vi "TCam_Overlay.vi"(8 "error in (no error)":errorcluster, 9 "OverlayTemp?":bool, 10 "Mouse pos":cluster{"X":i32, "Y":i32}, 11 "img in":T1) -> (0 "error out":errorcluster, 3 "Image Out":T1)   [LabVIEW 2024]
uses:
  <vilib>/vision/Image Controls.llb/IMAQ Image.ctl
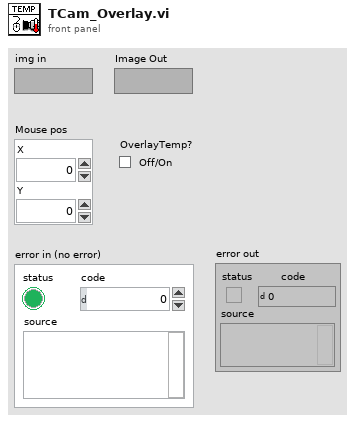
[diagram p1: front panel]
types:
  T1 = typedef "IMAQ Image.ctl" = refnum<image>
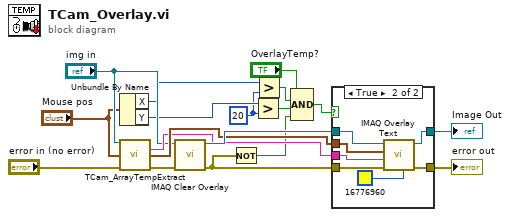
[diagram p0: block diagram]
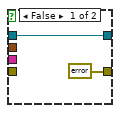
[diagram p2: hidden frame]
diagram:
  w3 = 20 ("x")
  n1 = Unbundle By Name("Mouse pos") -> ("X"=w2:i32, "Y"=w9:i32)
  n2 = call "TCam_ArrayTempExtract.vi"("img in"="img in", "Mouse pos"="Mouse pos", "error in (no error)"="error in (no error)") -> ("temp str"=w16:string, "Mouse pos dup"=w17:cluster{"X":i32, "Y":i32}, "error out"=w14:errorcluster)  [unwired: 8 in, 2 out]
  n3 = call "IMAQ Clear Overlay"("error in (no error)"=w14, "Image"="img in") -> ("error out"=w8:errorcluster, "Image Out"=w18:T1)  [unwired: 8 in]
  n4 = Not(x=w8) -> (.not. x?=w5:bool)
  n5 = Greater?(x=w9, y=w3) -> (0:w6:bool)
  n6 = Greater?(x=w2, y=w3) -> (0:w4:bool)
  n7 = Compound Arithmetic op=AND("OverlayTemp?", w4, w6, w5) -> (w7:bool)
  n8 = case shown="True" w7 {
    tunnel: w18 -> [w20 w27]
    tunnel: w8 -> [_ w26]
    tunnel: w17 -> [_ w25]
    tunnel: w16 -> [_ w24]
    tunnel: [w20 w23] -> w12
    tunnel: [errorcluster {"status"=FALSE, "code"=0, "source"=""} ("error out") w22] -> w11
    frame False {
    }
    frame True {
      n9 = call "IMAQ Overlay Text"("BG Color (Transparent)"=u32 16776960 ("Text Color (black)"), "error in (no error)"=w26, "String"=w24, "Origin"=w25, "Image"=w27) -> ("error out"=w22:errorcluster, "Image Out"=w23:T1)  [unwired: 5 in]
    }
  }
  "Image Out" <- w12
  "error out" <- w11
